vi "Play avi video.vi"() -> ()   [LabVIEW 2009]
panel:
  in  "AVI Path":path
  in  "stop":bool
  out "Image":T1(plugin-control)
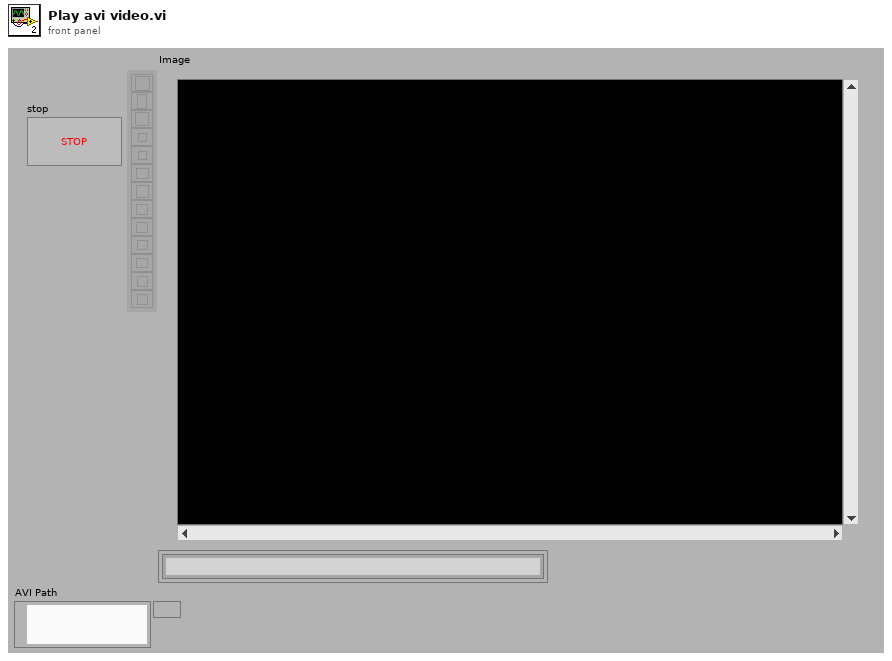
[diagram p1: front panel]
types:
  T1 = typedef "IMAQ Image.ctl" = refnum<image>
  T2 = typedef "AviRefnum.ctl" = refnum<k1>
  T3 = typedef "Image Type" = u32
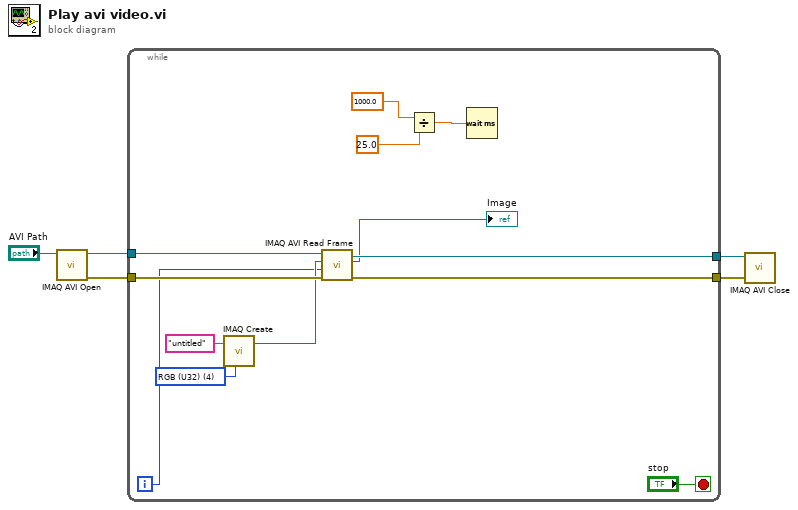
[diagram p0: block diagram]
diagram:
  n1 = call "IMAQ AVI Open"("AVI Path"="AVI Path") -> ("error out"=w3:errorcluster, "Avi Refnum"=w5:T2)  [unwired: 9 in]
  n2 = while {
    tunnel: w5 -> [w17]
    tunnel: [w16] -> w4
    tunnel: w3 -> [w15]
    tunnel: [w14] -> w2
    i -> [w11]
    stop <- "stop" stop-if-true
    w9 = T3 4 items=["Grayscale (U8)", "Grayscale (I16)", "Grayscale (SGL)", "Complex (CSG)", "RGB (U32)", "HSL (U32)", "RGB (U64)", "Grayscale (U16)"] ("Image Type")
    n3 = call "IMAQ Create"("Image Name"="untitled", "Image Type"=w9) -> ("New Image"=w12:T1)  [unwired: 3 in, 1 out]
    n4 = call "IMAQ AVI Read Frame"("error in (no error)"=w15, "Frame Number"=w11, "Image"=w12, "Avi Refnum"=w17) -> ("error out"=w14:errorcluster, "Image Out"=→"Image":T1, "Avi Refnum (duplicate)"=w16:T2)  [unwired: 4 in, 1 out]
    n5 = Divide(x=1000.0, y=25.0) -> (x/y=w8:dbl)
    n6 = Wait (ms)(milliseconds to wait=w8) -> ()  [unwired: 1 out]
  }
  n7 = call "IMAQ AVI Close"("error in (no error)"=w2, "Avi Refnum"=w4) -> ()  [unwired: 9 in, 1 out]
